vi "Formular.vi"() -> ()   [LabVIEW 2020]
panel:
  in  "m":dbl=30.0 format="%0.2f"
  in  "b":dbl=5.0 format="%0.2f"
  out "Waveform":dbl[][](graph)
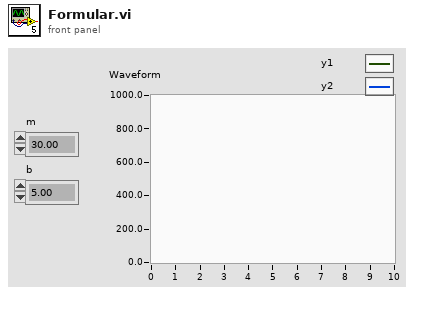
[diagram p1: front panel]
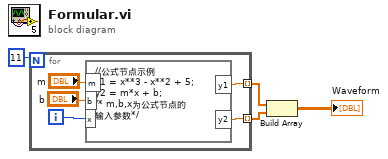
[diagram p0: block diagram]
diagram:
  n1 = for {
    N: 11 -> [_]
    tunnel: [w7] -> w2 mode=indexing
    tunnel: [w6] -> w1 mode=indexing
    i -> [w5]
    n2 = formula code="//公式节点示例\ny1 = x**3 - x**2 + 5;\ny2 = m*x + b;\n/* m,b,x为公式节点的\n输入参数*/"("m"="m", "b"="b", "x"=w5) -> ("y1"=w7:dbl, "y2"=w6:dbl)
  }
  n3 = Build Array "Build Array"(w2, w1) -> (→"Waveform":dbl[][])
